vi "CreatSaveITFile.vi"(8 "error in (no error)":errorcluster, 9 "index":i32, 11 "Data in":T1) -> (0 "error out":errorcluster, 1 "ITFileSave path":path, 3 "Data out":T1)   [LabVIEW 2014]
uses:
  controls/Data1.ctl
  controls/Payjson.ctl
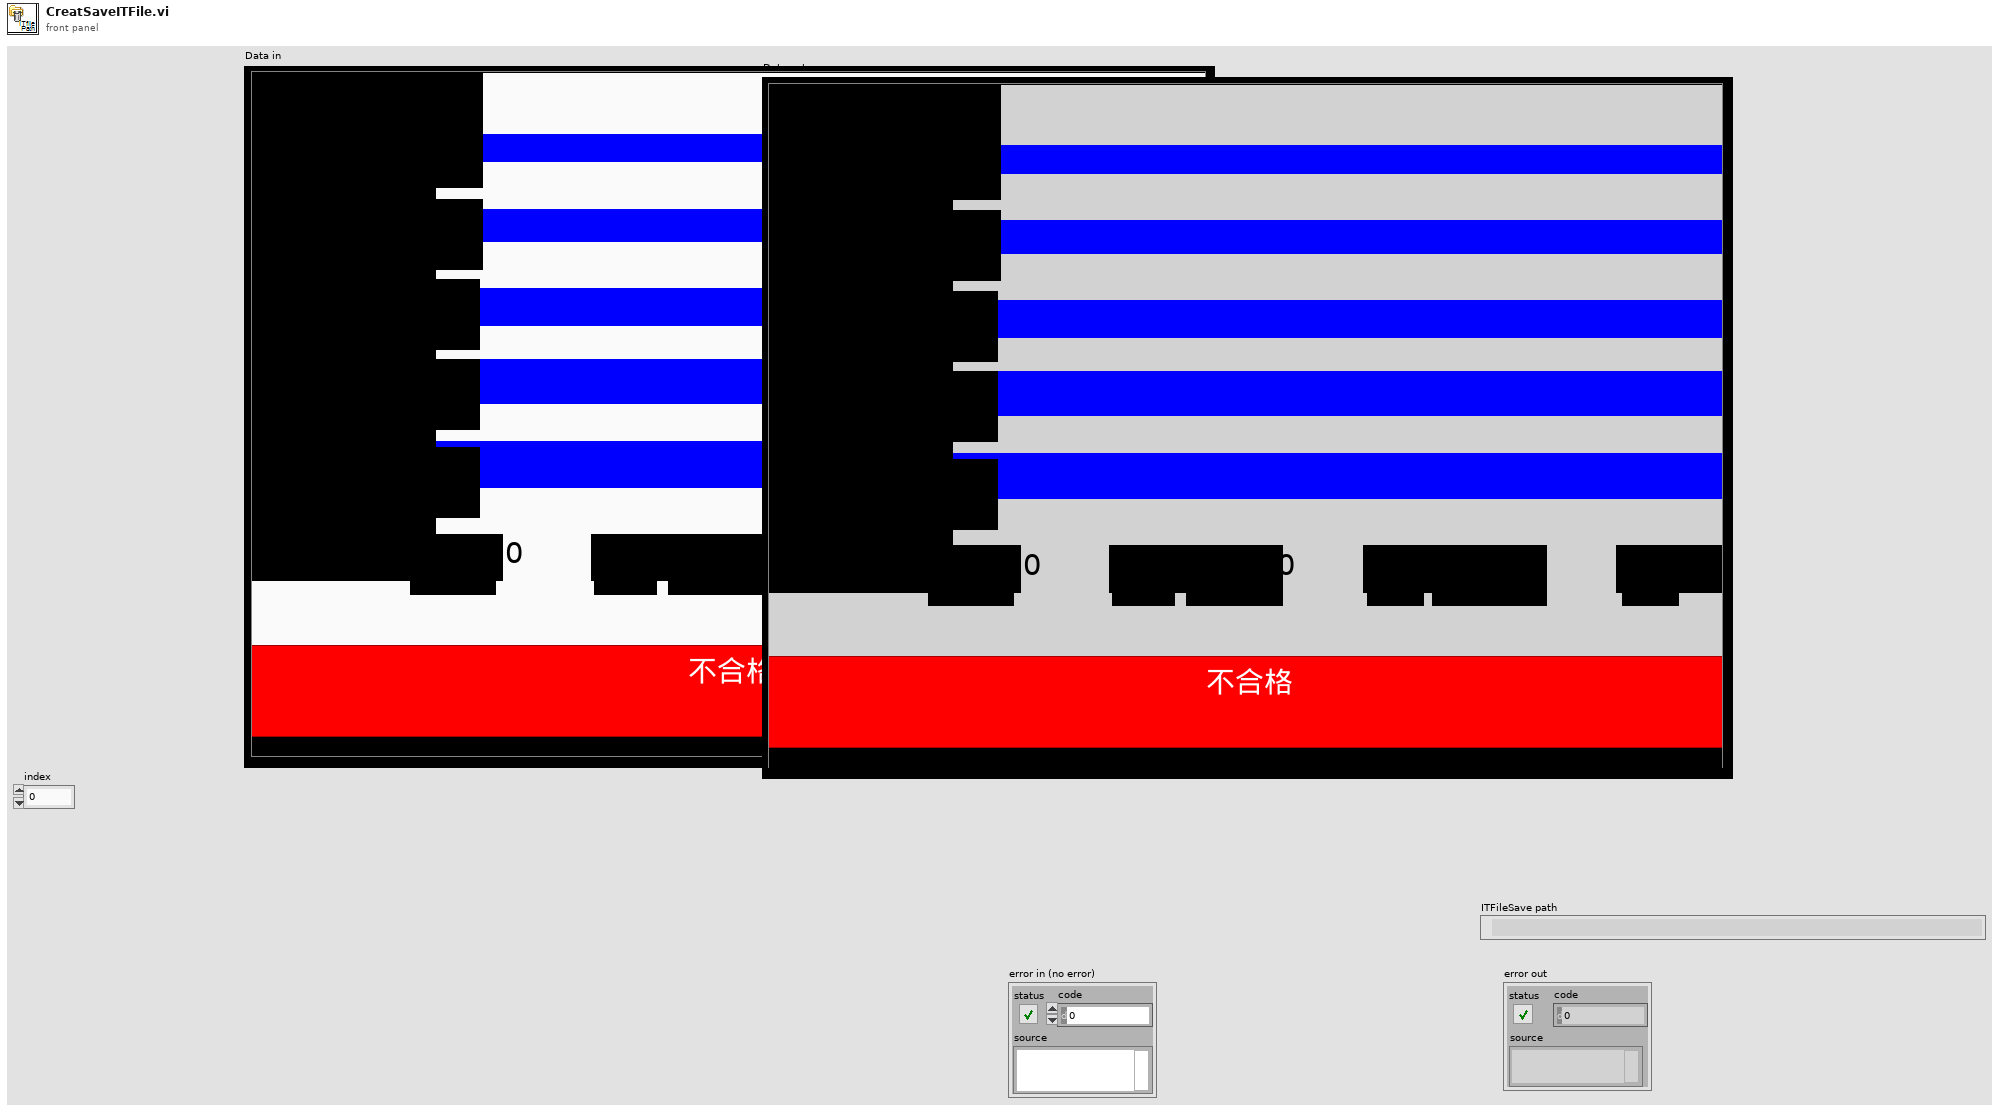
[diagram p1: front panel]
types:
  T1 = typedef "Data1.ctl" = cluster{"Date":string, "BarCode1":string, "BarCode2":string, "BarCode3":string, "Message":string, "OK Count":u16, "NG Count":u16, "Total Count":u16, "ModelData":string[][], "OK&NG":bool, "COM1":refnum<visa-resource-name>, "COM2":refnum<visa-resource-name>, "IO":i32, "Time":u32, "TCP":refnum<k5>, "TCP 2":refnum<k5>, "COM1 2":refnum<visa-resource-name>, "CheckNum":string, "BarCode1_1":string, "BarCode2_1":string, "BarCode3_1":string, "日期":string, "機種":string, "機號":string, "商品條碼1":string, "OK_1":string, "OK":string, "NG":string, "NG_1":string, "Total":string, "Total_1":string, "ClaerTime":u32, "Pjson":T2, "LotNo":string[], "CheckParsArray":string[], "BarCode4":string, "BarCode4_1":string, "商品條碼2":string, "BarCode5":string, "BarCode5_1":string, "商品條碼3":string, "ReScanNG":i32, "NGTimeCT":u32}
  T2 = typedef "Payjson.ctl" = cluster{"DEPT":string, "LINE":string, "STANO":string, "WORKNO":string, "PRODSN":string, "COMPNTID":string, "COMPNTLOT":string, "COMPNTSN":string, "USEDQTY":i16, "OPDATE":string, "OPUSER":string, "RECVDATE":string, "MMODU":string}[]
  T3 = cluster{"DEPT":string, "LINE":string, "STANO":string, "WORKNO":string, "PRODSN":string, "COMPNTID":string, "COMPNTLOT":string, "COMPNTSN":string, "USEDQTY":i16, "OPDATE":string, "OPUSER":string, "RECVDATE":string, "MMODU":string}
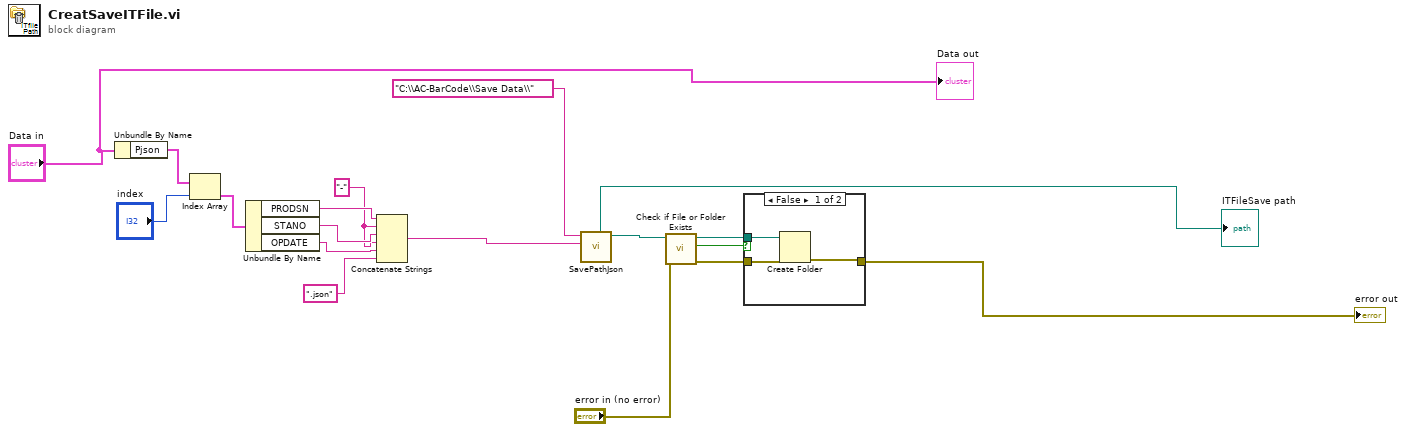
[diagram p0: block diagram]
diagram:
  w8 = "-" ("string")
  n1 = Unbundle By Name("Data in") -> ("Pjson"=w12:T2)
  n2 = Index Array(array=w12, index="index") -> (element=w11:T3)
  n3 = Unbundle By Name(w11) -> ("PRODSN"=w10:string, "STANO"=w9:string, "OPDATE"=w7:string)
  n4 = Concatenate Strings(w10, w8, w9, w8, w7, ".json" ("File Name")) -> (w5:string)
  n5 = call "SavePathJson.vi"("File Name"=w5, "Path In"="C:\\AC-BarCode\\Save Data\\") -> ("Folder Path"=w18:path, "File Path"=→"ITFileSave path":path)  [unwired: 8 in]
  n6 = call <vilib>:"Check if File or Folder Exists.vi"("error in (no error)"="error in (no error)", "path"=w18) -> ("error out"=w16:errorcluster, "file or folder exists?"=w17:bool, "dup path"=w15:path)  [unwired: 7 in]
  n7 = case shown="False" w17 {
    tunnel: w16 -> [w20 w22]
    tunnel: [w19 w22] -> w3
    tunnel: w15 -> [w21 _]
    frame False {
      n8 = Create Folder(path (use dialog)=w21, error in=w20) -> (error out=w19:errorcluster)  [unwired: 1 in, 2 out]
    }
    frame True {
    }
  }
  "error out" <- w3
  "Data out" <- "Data in"
